vi "HFRR ADV v05.vi"() -> ()   [LabVIEW 2025] (continued)
            n2842 = call "Instrument fgv.vi"("Enum"=T19."READ", "error in (no error) 2"=w3942, "INPUT"=w3940) -> ("error"=w3941:errorcluster, "output"=w3932:T13)  [unwired: 6 in, 1 out]
            n2843 = Bundle By Name(cluster=w3932, "String 36"="String") -> (w3931:T13)
            n2844 = case shown="True" "Write S" {
              selector: "Write S" -> [_ w3962]
              tunnel: w3941 -> [w3955 w3961]
              tunnel: [w3955 w3960] -> w3928
              tunnel: w3931 -> [w3954 w3957]
              tunnel: [w3954 w3956] -> w3927
              frame False {
              }
              frame True {
                n2845 = Not(x=w3962) -> (.not. x?=w3958:bool)
                n2846 = local write "Write S"(w3958) -> ()
                n2847 = call "Instrument fgv.vi"("Enum"=T19."MANUAL WRITE", "error in (no error) 2"=w3961, "INPUT"=w3957) -> ("error"=w3960:errorcluster, "output"=w3956:T13)  [unwired: 6 in, 1 out]
              }
            }
            n2848 = Array Size(array="WriteHumidity") -> (size(s)=w3925:i32)
            n2849 = Greater Than 0?(x=w3925) -> (x > 0?=w3923:bool)
            n2850 = call "Instrument fgv.vi"("Enum"=T19."WRITE", "error in (no error) 2"=w3928, "WriteCC1"="WriteHumidity", "INPUT"=w3927) -> ("error"=w3938:errorcluster, "WriteCC1 2"=w3926:string[], "output"=w3937:T13)  [unwired: 5 in]
            n2851 = case shown="True" w3923 {
              tunnel: w3926 -> [_ w3944]
              frame False {
              }
              frame True {
                n2852 = local write "WriteHumidity"(w3944) -> ()
              }
            }
            n2853 = case shown="Error" w3938 {
              selector: w3938 -> [w3945 w3948]
              tunnel: w3937 -> [w3946 w3953]
              tunnel: [w3946 w3952] -> w3935
              tunnel: [w3945 w3950] -> w3936
              frame No Error {
              }
              frame Error {
                n2854 = call <vilib>:"Clear Errors.vi"("error in (no error)"=w3948) -> ("error out"=w3947:errorcluster)  [unwired: 5 in, 1 out]
                n2855 = call "Instrument fgv.vi"("Enum"=T19."ERROR INIT", "error in (no error) 2"=w3947, "INPUT"=w3953) -> ("error"=w3951:errorcluster, "output"=w3952:T13)  [unwired: 6 in, 1 out]
                n2856 = call <vilib>:"Clear Errors.vi"("error in (no error)"=w3951) -> ("error out"=w3950:errorcluster)  [unwired: 5 in, 1 out]
              }
            }
            n2857 = Unbundle By Name(w3935) -> ("LastCom"=→"LastCom":string, "Read Heave and Surge"=→"Read Humidity":string)
          }
        }
        n2858 = Divide(x="Surge PPR", y="Surge Pitch") -> (x/y=→"Surge Pulses/mm":dbl)
        n2859 = Unbundle By Name(w3910) -> ("Heave COM Status 2"=w3912:bool, "Heave COM Status"=w3911:bool, "Error Heave"=w3908:errorcluster, "Bytes at Heave Port"=→"Bytes at Humidity Port":dbl)
        n2860 = Unbundle By Name(w3908) -> ("status"=→"Humidity Port":bool)
        n2861 = local write "Error Heave"(w3908) -> ()
        n2862 = Not(x=w3911) -> (.not. x?=w3896:bool)
        n2863 = Not(x=w3912) -> (.not. x?=w3897:bool)
        n2864 = local write "Instrument Status"(w3896) -> ()
        n2865 = local write "Heave COM Status 2"(w3897) -> ()
        n2866 = local read "Quit"() -> (w3889:bool)
        n2867 = Select(t=enum16{"init", "MAIN", "Panel Close"}."Panel Close", s=w3889, f=enum16{"init", "MAIN", "Panel Close"}."MAIN") -> (s? t:f=w3888:enum16{"init", "MAIN", "Panel Close"})
      }
      frame "Panel Close" {
      }
      frame Default {
      }
    }
  }
  n2868 = while {
    stop <- w3994 stop-if-true
    n2869 = local read "Read Humidity"() -> (w3972:string)
    n2870 = call <vilib>:"High Resolution Polling Wait.vi"("seconds to wait"=0.1) -> ()  [unwired: 10 in, 1 out]
    n2871 = String Length(string=w3972) -> (length=w3974:i32)
    n2872 = Less?(x=w3974, y=31 ("length")) -> (x < y?=w3970:bool)
    n2873 = case shown="False" w3970 {
      tunnel: w3972 -> [w3995 _]
      tunnel: [w3995 w3996] -> w3971
      frame False {
        "Read Humidity 2" <- w3995
      }
      frame True {
        n2874 = local read "Read Humidity 2"() -> (w3996:string)
      }
    }
    n2875 = Spreadsheet String To Array(delimiter (Tab)=",", format string="", spreadsheet string=w3971, array type (2D Dbl)=string[] []) -> (array=w3989:string[])
    n2876 = for {
      tunnel: w3989 -> [w3999] mode=indexing
      tunnel: string[] ["STATE;", "SET;", "RH;", "T;", "AMB_RH;", "AMB_T;", "PUMP;", "FAN_IN;", "FAN_OUT;", "DEHUM;", "CURRENT;", "STALL;"] -> [w3998] mode=indexing
      tunnel: [w3997] -> w3988 mode=indexing
      n2877 = Match Pattern(string=w3999, regular expression=w3998) -> (after substring=w3997:string)  [unwired: 1 in, 3 out]
    }
    n2878 = Index Array(array=w3988) -> (element #1=→"STATE :":string, element #2=→"SET :":string, element #3=w3977:string, element #4=→"T :":string, element #5=w3969:string, element #6=→"AMB_T :":string, element #7=→"PUMP :":string, element #8=→"FAN_IN :":string, element #9=→"FAN_OUT :":string, element #10=→"DEHUM :":string, element #11=→"CURRENT :":string, element #12=→"STALL :":string)  [unwired: 12 in]
    "RH :" <- w3977
    "AMB_RH :" <- w3969
    n2879 = Fract/Exp String To Number(string=w3977) -> (number=→"RH Numeric:":dbl)  [unwired: 3 in, 1 out]
    n2880 = Fract/Exp String To Number(string=w3969) -> (number=w3968:dbl)  [unwired: 3 in, 1 out]
    n2881 = local write "Ambient Humidity :"(w3968) -> ()
    n2882 = local read "Quit"() -> (w3994:bool)
  }
  n2883 = disable-structure shown="Disabled" {
    frame Disabled {
      n2884 = while {
        tunnel: [w4233] -> _
        i -> [w4233]
        stop <- w4230 stop-if-true
        n2885 = local read "powstat"() -> (w4231:bool)
        n2886 = case shown="True" w4231 {
          frame False {
          }
          frame True {
            n2887 = local read "RUN"() -> (w4234:bool)
            n2888 = case shown="True" w4234 {
              frame False {
                w4264 = 65.0 ("y")
                n2889 = local read "Set Hz"() -> (w4292:dbl)
                n2890 = local read "NORMAL LOAD"() -> (w4293:dbl)
                n2891 = Multiply(x=w4292, y=60.0) -> (x*y=w4299:dbl)
                n2892 = Multiply(x=1.2 ("y"), y=0.949) -> (x*y=w4268:dbl)
                n2893 = Multiply(x=1.2 ("y"), y=0.8166) -> (x*y=w4272:dbl)
                n2894 = Multiply(x=1.2 ("y"), y=0.851) -> (x*y=w4267:dbl)
                n2895 = local read "FF 2"() -> (w4291:dbl)
                n2896 = Absolute Value(x=w4299) -> (abs(x)=w4297:dbl)
                n2897 = local read "Stroke"() -> (w4266:dbl)
                n2898 = Less?(x=w4266, y=w4272) -> (x < y?=w4269:bool)
                n2899 = In Range and Coerce(upper limit=w4268, x=w4266, lower limit=w4267) -> (In Range?=w4270:bool)  [unwired: 1 out]
                n2900 = case shown="13.." w4291 {
                  tunnel: [1 2 3] -> w4289
                  frame 0..10, Default {
                    # "Normal"
                  }
                  frame 11, 12 {
                  }
                  frame 13.. {
                  }
                }
                "FF STATE" <- w4289
                n2901 = local read "TEMP"() -> (w4252:dbl)
                n2902 = case shown="3601.." w4297 {
                  tunnel: [1 2 3] -> w4295
                  frame 0..3000, Default {
                    # "Normal"
                  }
                  frame 3001..3600 {
                  }
                  frame 3601.. {
                  }
                }
                n2903 = case shown="11.." w4293 {
                  tunnel: [1 3] -> w4294
                  frame 1..10, Default {
                  }
                  frame 11.. {
                  }
                }
                "NL STATE" <- w4294
                n2904 = Multiply(x=1.2 ("y"), y=0.95) -> (x*y=w4282:dbl)
                n2905 = Multiply(x=w4264, y=0.954) -> (x*y=w4256:dbl)
                n2906 = Or(x=w4269, y=w4270) -> (x .or. y?=w4271:bool)
                n2907 = Greater Or Equal?(x=w4266, y=w4282) -> (x >= y?=w4279:bool)
                n2908 = Multiply(x=w4264, y=0.99) -> (x*y=w4253:dbl)
                n2909 = Greater Or Equal?(x=w4252, y=w4253) -> (x >= y?=w4258:bool)
                n2910 = Greater Or Equal?(x=w4252, y=w4256) -> (x >= y?=w4255:bool)
                n2911 = case shown="0, 1, Default" w4266 {
                  tunnel: [1 3] -> w4283
                  frame 0, 1, Default {
                  }
                  frame 2.. {
                  }
                }
                n2912 = case shown="True" w4279 {
                  tunnel: [1 3] -> w4284
                  frame False {
                  }
                  frame True {
                  }
                }
                n2913 = case shown="True" w4271 {
                  tunnel: [1 2] -> w4285
                  frame False {
                  }
                  frame True {
                  }
                }
                n2914 = case shown="..0" w4252 {
                  tunnel: [2 3 3 1] -> w4259
                  frame 61, 62 {
                  }
                  frame 63.. {
                  }
                  frame ..0 {
                  }
                  frame 10..60, Default {
                  }
                }
                n2915 = case shown="True" w4258 {
                  tunnel: [1 3] -> w4260
                  frame False {
                  }
                  frame True {
                  }
                }
                n2916 = Number To Decimal String(number=w4295) -> (decimal integer string=w4296:string)  [unwired: 1 in]
                n2917 = case shown="True" w4255 {
                  tunnel: [1 2] -> w4261
                  frame False {
                  }
                  frame True {
                  }
                }
                n2918 = Number To Decimal String(number=1) -> (decimal integer string=→"Air temp":string)  [unwired: 1 in]
                n2919 = Number To Decimal String(number=w4289) -> (decimal integer string=→"ff_st":string)  [unwired: 1 in]
                n2920 = local write "sp_st"(w4296) -> ()
                n2921 = Number To Decimal String(number=w4294) -> (decimal integer string=→"nl_st":string)  [unwired: 1 in]
                n2922 = Build Array(w4259, w4260, w4261) -> (w4262:i32[])
                n2923 = Build Array(w4283, w4284, w4285) -> (w4286:i32[])
                n2924 = Array Max & Min(array=w4262) -> (max value=w4263:i32)  [unwired: 3 out]
                n2925 = Array Max & Min(array=w4286) -> (max value=w4287:i32)  [unwired: 3 out]
                n2926 = Number To Decimal String(number=w4263) -> (decimal integer string=w4251:string)  [unwired: 1 in]
                n2927 = Number To Decimal String(number=w4287) -> (decimal integer string=→"Stroke Ln 2":string)  [unwired: 1 in]
                n2928 = local write "temp_st"(w4251) -> ()
              }
              frame True {
                w4349 = 65.0 ("y")
                # "Healthy -1\nWarning -2\nError -3"
                n2929 = local read "TEMP"() -> (w4360:dbl)
                n2930 = local read "NORMAL LOAD"() -> (w4364:dbl)
                n2931 = local read "Set Hz"() -> (w4362:dbl)
                n2932 = Multiply(x=1.2 ("y"), y=0.949) -> (x*y=w4344:dbl)
                n2933 = Multiply(x=1.2 ("y"), y=0.8166) -> (x*y=w4340:dbl)
                n2934 = Multiply(x=1.2 ("y"), y=0.851) -> (x*y=w4345:dbl)
                n2935 = Multiply(x=w4349, y=0.954) -> (x*y=w4356:dbl)
                n2936 = Multiply(x=w4349, y=0.99) -> (x*y=w4359:dbl)
                n2937 = Greater Or Equal?(x=w4360, y=w4359) -> (x >= y?=w4354:bool)
                n2938 = Multiply(x=w4362, y=60.0) -> (x*y=w4368:dbl)
                n2939 = Greater Or Equal?(x=w4360, y=w4356) -> (x >= y?=w4357:bool)
                n2940 = local read "FF 2"() -> (w4363:dbl)
                n2941 = local read "Stroke"() -> (w4346:dbl)
                n2942 = Less?(x=w4346, y=w4340) -> (x < y?=w4343:bool)
                n2943 = In Range and Coerce(upper limit=w4344, x=w4346, lower limit=w4345) -> (In Range?=w4342:bool)  [unwired: 1 out]
                n2944 = Absolute Value(x=w4368) -> (abs(x)=w4366:dbl)
                n2945 = case shown="63.." w4360 {
                  tunnel: [2 3 3 1] -> w4353
                  frame 61, 62 {
                  }
                  frame 63.. {
                  }
                  frame ..0 {
                  }
                  frame 10..60, Default {
                  }
                }
                n2946 = case shown="True" w4354 {
                  tunnel: [1 3] -> w4352
                  frame False {
                  }
                  frame True {
                  }
                }
                n2947 = case shown="True" w4357 {
                  tunnel: [1 2] -> w4351
                  frame False {
                  }
                  frame True {
                  }
                }
                n2948 = Multiply(x=1.2 ("y"), y=0.95) -> (x*y=w4330:dbl)
                n2949 = case shown="1..10, Default" w4364 {
                  tunnel: [1 3] -> w4371
                  frame 1..10, Default {
                  }
                  frame 11.. {
                  }
                }
                n2950 = case shown="0..10, Default" w4363 {
                  tunnel: [1 2 3] -> w4370
                  frame 0..10, Default {
                  }
                  frame 11, 12 {
                  }
                  frame 13.. {
                  }
                }
                n2951 = case shown="3601.." w4366 {
                  tunnel: [1 2 3] -> w4365
                  frame 0..3000, Default {
                    # "Normal"
                  }
                  frame 3001..3600 {
                  }
                  frame 3601.. {
                  }
                }
                n2952 = Or(x=w4343, y=w4342) -> (x .or. y?=w4341:bool)
                n2953 = Greater Or Equal?(x=w4346, y=w4330) -> (x >= y?=w4333:bool)
                n2954 = case shown="0, 1, Default" w4346 {
                  tunnel: [1 3] -> w4329
                  frame 0, 1, Default {
                  }
                  frame 2.. {
                  }
                }
                n2955 = case shown="True" w4333 {
                  tunnel: [1 3] -> w4328
                  frame False {
                  }
                  frame True {
                  }
                }
                n2956 = case shown="True" w4341 {
                  tunnel: [1 2] -> w4327
                  frame False {
                  }
                  frame True {
                  }
                }
                n2957 = Build Array(w4353, w4352, w4351) -> (w4350:i32[])
                n2958 = Number To Decimal String(number=w4365) -> (decimal integer string=→"sp_st":string)  [unwired: 1 in]
                n2959 = Array Max & Min(array=w4350) -> (max value=w4347:i32)  [unwired: 3 out]
                "TEMP STATE" <- w4347
                n2960 = Number To Decimal String(number=w4371) -> (decimal integer string=w4374:string)  [unwired: 1 in]
                n2961 = Number To Decimal String(number=w4370) -> (decimal integer string=w4372:string)  [unwired: 1 in]
                n2962 = Number To Decimal String(number=w4347) -> (decimal integer string=→"temp_st":string)  [unwired: 1 in]
                n2963 = Build Array(w4329, w4328, w4327) -> (w4326:i32[])
                n2964 = local write "nl_st"(w4374) -> ()
                n2965 = local write "ff_st"(w4372) -> ()
                n2966 = Number To Decimal String(number=1) -> (decimal integer string=w4369:string)  [unwired: 1 in]
                n2967 = Array Max & Min(array=w4326) -> (max value=w4325:i32)  [unwired: 3 out]
                n2968 = local write "Air temp"(w4369) -> ()
                n2969 = Number To Decimal String(number=w4325) -> (decimal integer string=w4324:string)  [unwired: 1 in]
                n2970 = local write "Stroke Ln 2"(w4324) -> ()
              }
            }
            n2971 = local read "Stroke Ln 2"() -> (w4236:string)
            n2972 = local read "nl_st"() -> (w4242:string)
            n2973 = local read "ff_st"() -> (w4239:string)
            n2974 = local read "sp_st"() -> (w4240:string)
            n2975 = local read "temp_st"() -> (w4241:string)
            n2976 = local read "Air temp"() -> (w4235:string)
            n2977 = Replace Array Subset(array="in", new element #1=w4242, index #1=1 ("index"), new element #2=w4239, index #2=2 ("index"), new element #3=w4241, index #3=3 ("index"), new element #4=w4240, index #4=4 ("index"), new element #5=w4236, index #5=5 ("index"), new element #6=w4235, index #6=6 ("index"), new element #7="Sensor State" ("new element/subarray"), index #7=0 ("index")) -> (→"out":string[])
          }
        }
        n2978 = Wait (ms)(milliseconds to wait=u32 10) -> ()  [unwired: 1 out]
        n2979 = local read "Quit"() -> (w4230:bool)
      }
      n2980 = while {
        stop <- w4205 stop-if-true
        n2981 = local read "run replace"() -> (w4207:bool)
        n2982 = Wait (ms)(milliseconds to wait=u32 100) -> ()  [unwired: 1 out]
        n2983 = Equal?(x="FLAG 2", y=0.0) -> (x = y?=w4208:bool)
        n2984 = case shown="True" w4208 {
          frame False {
          }
          frame True {
            n2985 = local write "FLAG 2"(100.0 ("FLAG 2")) -> ()
            n2986 = call <vilib>:"Read Characters From File.vi"("file path (dialog if empty)"=path "C:/LAB-IQ-NXT/WO 2449 TT.sig", "convert eol? (no:F)"=FALSE ("append to file? (new file:F)")) -> ("character string"=w4211:string)  [unwired: 4 in, 3 out]
            n2987 = call <vilib>:"Read Characters From File.vi"("file path (dialog if empty)"=path "C:/LAB-IQ-NXT/WO 2449 TRH.sig", "convert eol? (no:F)"=FALSE ("append to file? (new file:F)")) -> ("character string"=w4212:string)  [unwired: 4 in, 3 out]
            n2988 = Decimal String To Number(string=w4211) -> (number=w4213:i32)  [unwired: 2 in, 1 out]
            n2989 = local write "Total No. of Tests"(w4213) -> ()
            n2990 = Decimal String To Number(string=w4212) -> (number=w4216:i32)  [unwired: 2 in, 1 out]
            n2991 = local write "SEN.RUN HRS"(w4216) -> ()
          }
        }
        n2992 = case shown="True" w4207 {
          frame False {
          }
          frame True {
            n2993 = Equal?(x="FLAG 4", y=0.0) -> (x = y?=w4220:bool)
            n2994 = case shown="False" w4220 {
              frame False {
                n2995 = Get Date/Time In Seconds() -> (seconds since 1Jan1904=w4226:timestamp)
                n2996 = local read "START 3"() -> (w4224:dbl)
                n2997 = To Double Precision Float(number=w4226) -> (double precision float=w4225:dbl)
                n2998 = Subtract(x=w4225, y=w4224) -> (x-y=→"SENSOR TIME":dbl)
              }
              frame True {
                n2999 = Get Date/Time In Seconds() -> (seconds since 1Jan1904=w4228:timestamp)
                n3000 = local write "FLAG 4"(100.0 ("FLAG")) -> ()
                n3001 = To Double Precision Float(number=w4228) -> (double precision float=→"START 3":dbl)
              }
            }
          }
        }
        n3002 = local read "Quit"() -> (w4205:bool)
      }
      n3003 = while {
        shift-right: [w4005] -> _
        shift-left: _ -> [w4006]
        tunnel: [w4001] -> _
        i -> [w4001]
        stop <- w4000 stop-if-true
        n3004 = Wait (ms)(milliseconds to wait=u32 50 ("Refresh Rate (ms)")) -> ()  [unwired: 1 out]
        n3005 = local read "Json End Flg"() -> (w4002:bool)
        n3006 = Not(x="Upld AR 2") -> ()  [unwired: 1 out]
        n3007 = local read "Upld AR 2"() -> (w4003:bool)
        n3008 = call "Elapsed Time9"("Time Target (s)"="Sen.Upload Rate (s)", "Reset"=FALSE, "Auto Reset"=TRUE) -> ("Time has Elapsed"=w4012:bool)  [unwired: 9 in, 7 out]
        n3009 = Or(x=w4012, y=w4002) -> (x .or. y?=w4008:bool)
        n3010 = case shown="True" w4008 {
          frame False {
          }
          frame True {
            w4104 = "\"SensorName\":\"" ("string")
            w4074 = " \"},{"
            w4099 = "\",\"SensorState\":\""
            w4101 = "\",\"SensorModelNumber\":\"" ("string")
            w4100 = "\",\"SensorRuntimeHours\":\"" ("string")
            n3011 = local read "model num"() -> (w4098:string[])
            n3012 = local read "Sensor name"() -> (w4117:string[])
            n3013 = local read "run"() -> (w4088:string[])
            n3014 = local read "SENSOR TIME"() -> (w4044:dbl)
            n3015 = local read "out"() -> (w4037:string[])
            n3016 = local read "Total No. of Tests"() -> (w4042:dbl)
            n3017 = Select(t=60.0, s="Run test 3", f=3600.0) -> (s? t:f=w4052:dbl)
            n3018 = Index Array(array=w4098, index #1=1 ("index")) -> (element #1=w4097:string, element #2=w4096:string, element #3=w4095:string, element #4=w4094:string, element #5=w4093:string, element #6=w4092:string)  [unwired: 5 in]
            n3019 = Index Array(array=w4088, index #1=1 ("index")) -> (element #1=w4087:string, element #2=w4086:string, element #3=w4085:string, element #4=w4084:string, element #5=w4083:string, element #6=w4082:string)  [unwired: 5 in]
            n3020 = Index Array(array=w4117, index #1=1 ("index")) -> (element #1=w4116:string, element #2=w4115:string, element #3=w4114:string, element #4=w4113:string, element #5=w4103:string, element #6=w4102:string)  [unwired: 5 in]
            n3021 = Index Array(array=w4037, index #1=1 ("index")) -> (element #1=w4069:string, element #2=w4068:string, element #3=w4067:string, element #4=w4066:string, element #5=w4065:string, element #6=w4064:string)  [unwired: 5 in]
            n3022 = local read "SEN.RUN HRS"() -> (w4040:dbl)
            n3023 = Divide(x=w4044, y=w4052) -> (x/y=w4051:dbl)
            n3024 = Increment(x=w4051) -> (x+1=w4047:dbl)
            n3025 = Number To Decimal String(number=w4047) -> (decimal integer string=→"run hrs":string)  [unwired: 1 in]
            n3026 = Divide(x=w4040, y=3600.0 ("f")) -> (x/y=w4035:dbl)
            n3027 = Round To Nearest(number=w4035) -> (nearest integer value=w4033:dbl)
            n3028 = Number To Decimal String(number=w4033) -> (decimal integer string=w4034:string)  [unwired: 1 in]
            n3029 = Number To Decimal String(number=w4042) -> (decimal integer string=w4043:string)  [unwired: 1 in]
            n3030 = local read "Model No"() -> (w4048:string)
            n3031 = local read "UUID"() -> (w4143:string)
            n3032 = local read "Serial No"() -> (w4147:string)
            n3033 = local read "Secret Key"() -> (w4148:string)
            n3034 = Concatenate Strings("\",\"MachineSerialNumber\":\"" ("string"), w4147) -> (w4151:string)
            n3035 = Concatenate Strings("\",\"ModelNumber\":\"" ("string"), w4048) -> (w4049:string)
            n3036 = Concatenate Strings("\",\"MachineRuntimeHours\":\"" ("string"), w4034) -> (w4152:string)
            n3037 = Concatenate Strings("\",\"MachineRuntimeCycles\":\"", w4043) -> (w4145:string)
            n3038 = Concatenate Strings(w4101, w4097) -> (w4131:string)
            n3039 = Concatenate Strings(w4100, w4087) -> (w4132:string)
            n3040 = Concatenate Strings(w4099, w4069) -> (w4130:string)
            n3041 = Concatenate Strings(w4151, w4049, w4152, w4145) -> (w4154:string)
            n3042 = Concatenate Strings(w4101, w4096) -> (w4128:string)
            n3043 = Concatenate Strings(w4100, w4086) -> (w4127:string)
            n3044 = Concatenate Strings(w4099, w4068) -> (w4129:string)
            n3045 = Concatenate Strings(w4101, w4095) -> (w4123:string)
            n3046 = Concatenate Strings(w4100, w4085) -> (w4124:string)
            n3047 = Concatenate Strings(w4099, w4067) -> (w4122:string)
            n3048 = Concatenate Strings(w4101, w4094) -> (w4120:string)
            n3049 = Concatenate Strings(w4100, w4084) -> (w4119:string)
            n3050 = Concatenate Strings(w4099, w4066) -> (w4121:string)
            n3051 = Concatenate Strings(w4131, w4132, w4130) -> (w4133:string)
            n3052 = Concatenate Strings(w4101, w4093) -> (w4110:string)
            n3053 = Concatenate Strings(w4100, w4083) -> (w4111:string)
            n3054 = Concatenate Strings(w4101, w4092) -> (w4107:string)
            n3055 = Concatenate Strings(w4100, w4082) -> (w4106:string)
            n3056 = Concatenate Strings(w4099, w4065) -> (w4109:string)
            n3057 = Concatenate Strings(w4099, w4064) -> (w4108:string)
            n3058 = Concatenate Strings("{\"SecretKey\":\"", w4148, w4154, "\",\"UUID\" : \"", w4143, "\",\"SensorInformation\":", "[{" ("string")) -> (w4081:string)
            n3059 = Concatenate Strings(w4128, w4127, w4129) -> (w4126:string)
            n3060 = Concatenate Strings(w4123, w4124, w4122) -> (w4125:string)
            n3061 = Concatenate Strings(w4120, w4119, w4121) -> (w4118:string)
            n3062 = Concatenate Strings(w4110, w4111, w4109) -> (w4112:string)
            n3063 = Concatenate Strings(w4107, w4106, w4108) -> (w4105:string)
            n3064 = Concatenate Strings(w4104, w4116, w4133, w4074) -> (w4080:string)
            n3065 = Concatenate Strings(w4104, w4115, w4126, w4074) -> (w4079:string)
            n3066 = Concatenate Strings(w4104, w4114, w4125, w4074) -> (w4078:string)
            n3067 = Concatenate Strings(w4104, w4113, w4118, w4074) -> (w4077:string)
            n3068 = Concatenate Strings(w4104, w4103, w4112, w4074) -> (w4076:string)
            n3069 = Concatenate Strings(w4104, w4102, w4105, "\"}" ("string")) -> (w4075:string)
            n3070 = Concatenate Strings(w4081, w4080, w4079, w4078, w4077, w4076, w4075, "]}" ("string")) -> (w4072:string)
            n3071 = local read "SEN.RUN HRS"() -> (w4039:dbl)
            n3072 = disable-structure shown="Disabled" {
              frame Disabled {
                n3073 = local read "state"() -> (w4158:string[])
                n3074 = Delete From Array(array=w4158, index=0) -> (array with subset deleted=w4156:string[])  [unwired: 1 in, 1 out]
                n3075 = for {
                  N: 6 -> [_]
                  tunnel: w4156 -> [w4169] mode=indexing
                  tunnel: [w4168] -> w4155 mode=indexing
                  n3076 = Equal?(x=w4169, y="Warning") -> (x = y?=w4165:bool)
                  n3077 = Equal?(x=w4169, y="Healthy") -> (x = y?=w4162:bool)
                  n3078 = Select(t="2" ("y"), s=w4165, f="3" ("y")) -> (s? t:f=w4160:string)
                  n3079 = Select(t="1" ("y"), s=w4162, f=w4160) -> (s? t:f=w4168:string)
                }
                "state1" <- w4155
              }
              frame Enabled {
              }
            }
            n3080 = stacked-sequence {
              tunnel: w4072 -> [w4180 _ _]
              tunnel: [_ _ w4196] -> _
              frame #0 {
                (unwired) FALSE ("convert eol (F)")
                w4182 = enum16{"start", "end", "current"}."start" ("pos mode (0:2)")
                n3081 = local read "Path"() -> (w4176:path)
                n3082 = Path To String(path=w4176) -> (string=w4188:string)
                n3083 = Concatenate Strings(w4188, "\\", "Sensor File Name") -> (w4189:string)
                n3084 = local write "standard output 2"(" ") -> ()
                n3085 = String To Path(string=w4189) -> (path=w4179:path)
                n3086 = call <vilib>:"Open_Create_Replace File.vi"("advisory dialog? (display:T)"=FALSE, "function (open:0)"=T20."create or replace", "file path"=w4179) -> ("error out"=w4192:errorcluster, "refnum"=w4191:refnum<file>)  [unwired: 5 in, 2 out]
                n3087 = Set File Position(refnum=w4191, from (0:start)=w4182, error in=w4192) -> (refnum out=w4172:refnum<file>, error out=w4171:errorcluster)  [unwired: 1 in]
                n3088 = Write to Binary File(file (use dialog)=w4172, data=" ", error in=w4171, 5:FALSE ("prepend array or string size? (T)")) -> (refnum out=w4183:refnum<file>, error out=w4184:errorcluster)  [unwired: 2 in, 1 out]
                n3089 = Set File Position(offset (in bytes) (0)=w4182, refnum=w4183, error in=w4184) -> (refnum out=w4175:refnum<file>, error out=w4174:errorcluster)  [unwired: 1 in]
                n3090 = Write to Binary File(file (use dialog)=w4175, data=w4180, error in=w4174, 5:FALSE ("prepend array or string size? (T)")) -> (error out=w4178:errorcluster)  [unwired: 2 in, 2 out]
                n3091 = flat-sequence {
                  tunnel: w4179 -> [w4194]
                  tunnel: w4178 -> [_]
                  frame #0 {
                    n3092 = call <vilib>:"Read Characters From File.vi"("file path (dialog if empty)"=w4194) -> ("character string"=→"Sensor Health JSON string":string)  [unwired: 5 in, 3 out]
                  }
                }
                "SinglePoint  2" <- w4180
              }
              frame #1 {
              }
              frame #2 {
                (unwired) "\"Stored\": true" ("string")
                n3093 = call <vilib>:"System Exec.vi"("run minimized? (F)"=TRUE, "wait until completion? (T)"=TRUE, "working directory"=path "C:/LAB-IQ-NXT", "command line"="C:\\LAB-IQ-NXT\\JPostH.bat") -> ("standard error"=→"Respose From Server 2":string, "standard output"=w4199:string)  [unwired: 4 in, 2 out]
                "standard output 2" <- w4199
                n3094 = Match Pattern(string=w4199, regular expression="JSONH Check String") -> (match substring=w4197:string, offset past match=w4196:i32)  [unwired: 1 in, 2 out]
                n3095 = Equal?(x=w4197, y="JSONH Check String") -> (x = y?=→"Upload \nConfirmed 2":bool)
              }
            }
            n3096 = Divide(x=w4039, y=3600.0 ("f")) -> (x/y=w4032:dbl)
            n3097 = local read "run time"() -> (w4089:string[])
            n3098 = Round To Nearest(number=w4032) -> (nearest integer value=w4031:dbl)
            n3099 = Number To Decimal String(number=w4031) -> (decimal integer string=w4030:string)  [unwired: 1 in]
            n3100 = Index Array(array="Sensor Information", index (col) #1=0 ("disabled index (col)"), index (col) #2=1 ("index (col)"), index (col) #3=2 ("index (col)"), index (col) #4=3 ("index (col)")) -> (element #1=→"Sensor name":string[], element #2=→"model num":string[], element #3=→"run time":string[], element #4=→"state":string[])  [unwired: 4 in]
            n3101 = Insert Into Array(array=w4089, index=1, new element #1=w4030, new element #2=w4030, new element #3=w4030, new element #4=w4030, new element #5=w4030, new element #6=w4030) -> (w4054:string[])
            "run" <- w4054
            n3102 = local read "out"() -> (w4036:string[])
            n3103 = local read "Sensor Information"() -> (w4056:string[][])
            n3104 = Replace Array Subset(array=w4056, new element #1=w4054, index (col) #1=2 ("disabled index (col)"), new element #2=w4036, index (col) #2=3 ("index (col)")) -> (w4055:string[][])  [unwired: 2 in]
            n3105 = local write "Sensor Information"(w4055) -> ()
          }
        }
        n3106 = case shown="True" w4003 {
          frame False {
          }
          frame True {
            n3107 = Equal?(x="FLAG", y=0.0) -> (x = y?=w4020:bool)
            n3108 = case shown="False" w4020 {
              frame False {
                n3109 = Get Date/Time In Seconds() -> (seconds since 1Jan1904=w4026:timestamp)
                n3110 = local read "START 2"() -> (w4024:dbl)
                n3111 = To Double Precision Float(number=w4026) -> (double precision float=w4025:dbl)
                n3112 = Subtract(x=w4025, y=w4024) -> (x-y=→"SENSOR TIME  2":dbl)
              }
              frame True {
                n3113 = Get Date/Time In Seconds() -> (seconds since 1Jan1904=w4028:timestamp)
                n3114 = To Double Precision Float(number=w4028) -> (double precision float=→"START 2":dbl)
                n3115 = local write "FLAG"(100.0 ("FLAG")) -> ()
              }
            }
          }
        }
        n3116 = disable-structure shown="Disabled" {
          disable-tunnel: w4006 -> [w4015 _]
          disable-tunnel: [w4014 _] -> w4005
          frame Disabled {
            n3117 = local read "Json St Flg"() -> (w4013:bool)
            n3118 = case shown="True" w4013 {
              tunnel: w4015 -> [w4016 w4018]
              tunnel: [w4016 w4017] -> w4014
              frame False {
              }
              frame True {
                n3119 = Increment(x=w4018) -> (x+1=w4017:dbl)
                "T cycle" <- w4017
                n3120 = local write "Json St Flg"(FALSE ("Json St Flg")) -> ()
              }
            }
          }
          frame Enabled {
          }
        }
        n3121 = local read "Quit"() -> (w4000:bool)
      }
    }
    frame Enabled {
    }
  }
  n3122 = stacked-sequence {
    tunnel: [w4398] -> w18
    frame #0 {
      w4398 = FALSE ("Upload \nConfirmed")
      n3123 = local write "Upload \nConfirmed"(w4398) -> ()
      n3124 = local write "St Str"("") -> ()
    }
  }
  n3125 = disable-structure shown="Disabled" {
    disable-tunnel: w18 -> [w4399 _]
    frame Disabled {
      n3126 = case shown="True" {
        selector: _ -> [_ _]
        tunnel: w4399 -> [_ w4400]
        frame False {
        }
        frame True {
          n3127 = while {
            tunnel: [w4406] -> _
            tunnel: w4400 -> [_]
            i -> [w4406]
            stop <- w4401 stop-if-true
            n3128 = local read "Json End Flg"() -> (w4405:bool)
            n3129 = Wait (ms)(milliseconds to wait=u32 20 ("Refresh Rate (ms)")) -> ()  [unwired: 1 out]
            n3130 = local read "refresh flag"() -> (w4402:bool)
            n3131 = local read "RUN"() -> (w4403:bool)
            n3132 = And(x=w4403, y=w4402) -> (x .and. y?=w4404:bool)
            n3133 = Or(x=w4404, y=w4405) -> (x .or. y?=w4407:bool)
            "AR Led" <- w4407
            n3134 = case shown="True" w4407 {
              frame False {
              }
              frame True {
                w4424 = "\",\""
                n3135 = local read "UUID"() -> (w4422:string)
                n3136 = local write "refresh flag"(FALSE ("refresh flag")) -> ()
                n3137 = local read "time"() -> (w4411:dbl)
                n3138 = Multiply(x=w4411, y=60.0) -> (x*y=w4410:dbl)
                n3139 = Concatenate Strings("UUID\" : \"", w4422, "\"}") -> (w4425:string)
                n3140 = Number To Fractional String(number=w4410, width (-)=i16 10, precision (6)=i16 4) -> (F-format string=w4439:string)  [unwired: 1 in]
                n3141 = Concatenate Strings("{", "\"Time\":\"", w4439, w4424) -> (w4434:string)
                n3142 = stacked-sequence {
                  tunnel: w4424 -> [w4487 w4495 w4502 w4510 w4518 w4527 w4534]
                  tunnel: [w4488 _ _ _ _ _ _] -> w4438
                  tunnel: [_ w4496 _ _ _ _ _] -> w4437
                  tunnel: [_ _ w4503 _ _ _ _] -> w4436
                  tunnel: [_ _ _ w4512 _ _ _] -> w4435
                  tunnel: w4425 -> [_ _ _ _ _ _ w4545]
                  tunnel: [_ _ _ _ _ _ w4544] -> w4421
                  tunnel: [_ _ _ _ _ w4524 _] -> w4420
                  tunnel: [_ _ _ _ w4517 _ _] -> w4419
                  frame #0 {
                    n3143 = local read "NORMAL LOAD"() -> (w4486:dbl)
                    n3144 = Number To Fractional String(number=w4486, width (-)=i16 10, precision (6)=i16 4) -> (F-format string=w4489:string)  [unwired: 1 in]
                    n3145 = Concatenate Strings("NormalLoad\":\"", w4489, w4487) -> (w4488:string)
                  }
                  frame #1 {
                    n3146 = local read "Temp"() -> (w4494:dbl)
                    n3147 = Number To Fractional String(number=w4494, width (-)=i16 10, precision (6)=i16 4) -> (F-format string=w4497:string)  [unwired: 1 in]
                    n3148 = Concatenate Strings("Temperature\":\"", w4497, w4495) -> (w4496:string)
                  }
                  frame #2 {
                    n3149 = local read "cof"() -> (w4500:dbl)
                    n3150 = Number To Fractional String(number=w4500, width (-)=i16 10, precision (6)=i16 4) -> (F-format string=w4504:string)  [unwired: 1 in]
                    n3151 = Concatenate Strings("FrictionalForce\":\"", w4504, w4502) -> (w4503:string)
                  }
                  frame #3 {
                    n3152 = local read "Set Hz"() -> (w4508:dbl)
                    n3153 = Multiply(x=w4508, y=60.0) -> (x*y=w4507:dbl)
                    n3154 = Number To Fractional String(number=w4507, width (-)=i16 10, precision (6)=i16 4) -> (F-format string=w4513:string)  [unwired: 1 in]
                    n3155 = Concatenate Strings("Speed\":\"", w4513, w4510) -> (w4512:string)
                  }
                  frame #4 {
                    n3156 = local read "Stroke Ln"() -> (w4516:dbl)
                    n3157 = Number To Fractional String(number=w4516, width (-)=i16 10, precision (6)=i16 4) -> (F-format string=w4520:string)  [unwired: 1 in]
                    n3158 = Concatenate Strings("LinearDeformation\":\"", w4520, w4518) -> (w4517:string)
                  }
                  frame #5 {
                    n3159 = local read "AIR TEMP"() -> (w4523:dbl)
                    n3160 = local read "Json St Flg"() -> (w4525:bool)
                    n3161 = local read "Json End Flg"() -> (w4526:bool)
                    n3162 = Number To Fractional String(number=w4523, width (-)=i16 10, precision (6)=i16 4) -> (F-format string=w4529:string)  [unwired: 1 in]
                    n3163 = Concatenate Strings("Vibration\":\"", w4529, w4527) -> (w4524:string)
                    n3164 = And(x=w4525, y=w4526) -> ()  [unwired: 1 out]
                  }
                  frame #6 {
                    n3165 = local read "Json End Flg"() -> (w4533:bool)
                    n3166 = Get Date/Time In Seconds() -> (seconds since 1Jan1904=w4541:timestamp)
                    n3167 = local read "Json St Flg"() -> (w4532:bool)
                    n3168 = To Double Precision Float(number=w4541) -> (double precision float=w4540:dbl)
                    n3169 = Subtract(x=w4540, y=2082844800.0) -> (x-y=w4538:dbl)
                    n3170 = Number To Fractional String(number=w4538, width (-)=i16 12, precision (6)=i16 0) -> (F-format string=w4535:string)  [unwired: 1 in]
                    n3171 = case shown="True" w4533 {
                      tunnel: ["" w4548] -> w4542
                      tunnel: w4535 -> [_ w4549]
                      tunnel: w4534 -> [_ w4547]
                      frame False {
                      }
                      frame True {
                        n3172 = local write "Json End Flg"(FALSE ("Json St Flg")) -> ()
                        n3173 = Concatenate Strings("End\": \"", w4549, w4547) -> (w4548:string)
                      }
                    }
                    n3174 = case shown="True" w4532 {
                      tunnel: [w4552 w4555] -> w4543
                      tunnel: w4535 -> [_ w4556]
                      tunnel: w4534 -> [_ w4553]
                      frame False {
                        n3175 = local read "St Str"() -> (w4552:string)
                      }
                      frame True {
                        n3176 = Concatenate Strings("Start\":\"", w4556, w4553) -> (w4555:string)
                        "St Str" <- w4555
                        n3177 = local write "Json St Flg"(FALSE ("Json St Flg")) -> ()
                      }
                    }
                    n3178 = Concatenate Strings(w4543, w4542, w4545) -> (w4544:string)
                  }
                }
                n3179 = local read "FILE"() -> (w4413:string)
                n3180 = Concatenate Strings("\",\"OperatorID\":\"" ("string"), "Operator ID") -> (w4416:string)
                n3181 = Concatenate Strings("\",\"DatasetTitle\":\"" ("string"), w4413) -> (w4415:string)
                n3182 = Concatenate Strings("\",\"SerialNumber\":\"" ("string"), "Serial No") -> (w4445:string)
                n3183 = Concatenate Strings("\",\"ModelNumber\":\"" ("string"), "Model No") -> (w4444:string)
                n3184 = Concatenate Strings(w4445, w4444) -> (w4427:string)
                n3185 = Concatenate Strings("{\"SecretKey\":\"", "Secret Key", w4427, w4416, w4415, "\",\"Samples\":[") -> (w4432:string)
                n3186 = Concatenate Strings(w4434, w4438, w4437, w4436, w4435, w4419, w4420, w4421) -> (w4433:string)
                n3187 = Concatenate Strings(w4432, w4433, "]}") -> (w4431:string)
                n3188 = stacked-sequence {
                  tunnel: w4431 -> [w4460 _ _]
                  tunnel: [_ _ w4477] -> _
                  frame #0 {
                    (unwired) FALSE ("convert eol (F)")
                    w4462 = enum16{"start", "end", "current"}."start" ("pos mode (0:2)")
                    n3189 = Path To String(path="Path") -> (string=w4468:string)
                    n3190 = Concatenate Strings(w4468, "\\", "Data File Name") -> (w4470:string)
                    n3191 = local write "standard output"(" ") -> ()
                    n3192 = String To Path(string=w4470) -> (path=w4459:path)
                    n3193 = call <vilib>:"Open_Create_Replace File.vi"("advisory dialog? (display:T)"=FALSE, "function (open:0)"=T20."create or replace", "file path"=w4459) -> ("error out"=w4473:errorcluster, "refnum"=w4472:refnum<file>)  [unwired: 5 in, 2 out]
                    n3194 = Set File Position(refnum=w4472, from (0:start)=w4462, error in=w4473) -> (refnum out=w4453:refnum<file>, error out=w4452:errorcluster)  [unwired: 1 in]
                    n3195 = Write to Binary File(file (use dialog)=w4453, data=" ", error in=w4452, 5:FALSE ("prepend array or string size? (T)")) -> (refnum out=w4463:refnum<file>, error out=w4464:errorcluster)  [unwired: 2 in, 1 out]
                    n3196 = Set File Position(offset (in bytes) (0)=w4462, refnum=w4463, error in=w4464) -> (refnum out=w4456:refnum<file>, error out=w4455:errorcluster)  [unwired: 1 in]
                    n3197 = Write to Binary File(file (use dialog)=w4456, data=w4460, error in=w4455, 5:FALSE ("prepend array or string size? (T)")) -> (error out=w4458:errorcluster)  [unwired: 2 in, 2 out]
                    n3198 = flat-sequence {
                      tunnel: w4459 -> [w4475]
                      tunnel: w4458 -> [_]
                      frame #0 {
                        n3199 = call <vilib>:"Read Characters From File.vi"("file path (dialog if empty)"=w4475) -> ("character string"=→"JSON string":string)  [unwired: 5 in, 3 out]
                      }
                    }
                    "SinglePoint" <- w4460
                  }
                  frame #1 {
                  }
                  frame #2 {
                    (unwired) "\"Stored\": true" ("string")
                    n3200 = call <vilib>:"System Exec.vi"("run minimized? (F)"=TRUE, "wait until completion? (T)"=TRUE, "working directory"=path "C:/LAB-IQ-NXT", "command line"="C:\\LAB-IQ-NXT\\JPost.bat") -> ("standard error"=→"Respose From Server":string, "standard output"=w4480:string)  [unwired: 4 in, 2 out]
                    "standard output" <- w4480
                    n3201 = Match Pattern(string=w4480, regular expression="JSON Check String") -> (match substring=w4478:string, offset past match=w4477:i32)  [unwired: 1 in, 2 out]
                    n3202 = Equal?(x=w4478, y="JSON Check String") -> (x = y?=→"Upload \nConfirmed":bool)
                  }
                }
              }
            }
            n3203 = local read "Quit"() -> (w4401:bool)
          }
        }
      }
    }
    frame Enabled {
    }
  }
  n3204 = disable-structure shown="Disabled" {
    disable-tunnel: w17 -> [w4563 _]
    frame Disabled {
      n3205 = while {
        shift-right: [w4571] -> w4559
        shift-left: _ -> [w4572]
        shift-right: [w4569] -> w4560
        shift-left: errorcluster {"status"=TRUE, "code"=0, "source"="Init"} ("error out") -> [w4570]
        shift-right: [w4567] -> _
        shift-left: "" -> [w4568]
        tunnel: [w4565] -> _
        tunnel: w4563 -> [_]
        i -> [w4565]
        stop <- w4564 stop-if-true
        n3206 = flat-sequence {
          tunnel: [w4573] -> w4566
          frame #0 {
            n3207 = Wait (ms)(milliseconds to wait=10.0 ("Delay")) -> (millisecond timer value=w4573:u32)
          }
        }
        n3208 = case shown="No Error" w4570 {
          selector: w4570 -> [w4606 w4728]
          tunnel: [w4588 w4730] -> w4571
          tunnel: [w4587 w4729] -> w4569
          tunnel: w4572 -> [w4607 w4722]
          tunnel: w4568 -> [w4586 w4721]
          tunnel: [w4585 w4721] -> w4567
          tunnel: w4566 -> [_ _]
          frame No Error {
            n3209 = Concatenate Strings("COMMAND", "\r", "\n") -> (w4597:string)
            n3210 = case shown="True" "Measure" {
              tunnel: w4607 -> [w4633 w4640]
              tunnel: w4606 -> [w4632 w4639]
              tunnel: [w4633 w4638] -> w4605
              tunnel: [w4632 w4637] -> w4584
              tunnel: w4597 -> [_ w4636]
              frame False {
              }
              frame True {
                n3211 = VISA Write(VISA resource name=w4640, write buffer=w4636, error in (no error)=w4639) -> (VISA resource name out=w4638:refnum<visa-resource-name>, error out=w4637:errorcluster)  [unwired: 1 out]
                n3212 = local write "Read String"("") -> ()
                n3213 = local write "Measure"(FALSE) -> ()
              }
            }
            n3214 = property class="Instr"(reference=w4605, error in=w4584) -> (reference out=w4604:refnum<visa-resource-name>, error out=w4603:errorcluster, "Serial Settings:Number of Bytes at Serial Port"=w4602:u32)
            n3215 = Greater?(x=w4602, y=u32 100) -> (0:w4600:bool)
            n3216 = case shown="True" w4600 {
              tunnel: w4604 -> [w4643 w4668]
              tunnel: w4603 -> [w4642 w4667]
              tunnel: w4602 -> [_ w4666]
              tunnel: [w4643 w4665] -> w4590
              tunnel: [w4642 w4664] -> w4589
              tunnel: w4586 -> [w4641 w4663]
              tunnel: [w4641 ""] -> w4585
              frame False {
              }
              frame True {
                w4653 = u32 6 ("y")
                # "Page 84 of \nmanual"
                n3217 = VISA Read(VISA resource name=w4668, byte count=w4666, error in (no error)=w4667) -> (VISA resource name out=w4665:refnum<visa-resource-name>, read buffer=w4661:string, error out=w4664:errorcluster)  [unwired: 1 out]
                n3218 = while {
                  tunnel: w4661 -> [w4717]
                  tunnel: [w4713] -> w4655 mode=indexing
                  tunnel: [w4707] -> w4659 mode=indexing
                  tunnel: [w4705] -> _
                  i -> [w4705]
                  stop <- w4710 stop-if-true
                  n3219 = String Subset(string=w4717, offset (0)=w4705) -> (substring=w4712:string)  [unwired: 1 in]
                  n3220 = String To Byte Array(string=w4712) -> (unsigned byte array=w4716:u8[])
                  n3221 = String Length(string=w4712) -> (length=w4711:i32)
                  n3222 = Index Array(array=w4716) -> (element=w4715:u8)  [unwired: 1 in]
                  n3223 = Equal To 0?(x=w4711) -> (x = 0?=w4710:bool)
                  n3224 = Number To Boolean Array(number=w4715) -> (Boolean array=w4709:bool[])
                  n3225 = Reverse 1D Array(array=w4709) -> (reversed array=w4708:bool[])
                  n3226 = And(x=w4709, y=bool[] [FALSE, FALSE, FALSE, FALSE, FALSE, FALSE, TRUE, TRUE] ("Boolean array")) -> (x .and. y?=w4713:bool[])
                  n3227 = And(x=w4708, y=bool[] [FALSE, FALSE, TRUE, TRUE, TRUE, TRUE, TRUE, TRUE] ("Boolean array")) -> (x .and. y?=w4707:bool[])
                }
                n3228 = Concatenate Strings(w4663, w4661) -> (→"Read String":string)
                n3229 = while {
                  tunnel: w4655 -> [w4704] mode=indexing
                  tunnel: [w4700] -> w4658
                  i -> [w4700]
                  stop <- w4701 stop-if-true
                  n3230 = Search 1D Array(1D array=w4704, element=TRUE) -> (index of element=w4702:i32)  [unwired: 1 in]
                  n3231 = Less Than 0?(x=w4702) -> (x < 0?=w4701:bool)
                }
                n3232 = Delete From Array(array=w4659, length=w4658, index (row)=0) -> (array with subset deleted=w4654:bool[][])  [unwired: 1 in, 1 out]
                n3233 = Array Size(array=w4654) -> (size(s)=w4656:i32[])
                n3234 = Index Array(array=w4656) -> (element=w4648:i32)  [unwired: 1 in]
                n3235 = Greater?(x=w4648, y=w4653) -> (0:w4651:bool)
                n3236 = Subtract(x=w4648, y=w4653) -> (x-y=w4652:u32)
                n3237 = Select(t=w4652, s=w4651, f=u32 0) -> (s? t:f=w4649:u32)
                n3238 = while {
                  tunnel: w4654 -> [w4687]
                  tunnel: [w4689] -> w4647 mode=indexing
                  tunnel: w4649 -> [w4671]
                  i -> [w4688]
                  stop <- w4686 stop-if-true
                  w4678 = 6 ("index")
                  w4677 = 2 ("length")
                  # "Page 65 of \nmanual"
                  n3239 = Multiply(x=u32 3 ("y"), y=w4688) -> (x*y=w4685:u32)
                  n3240 = Divide(x=u32 102 ("y"), y=u32 65520) -> (x/y=w4695:dbl)
                  n3241 = Greater Or Equal?(x=w4685, y=w4671) -> (x >= y?=w4686:bool)
                  n3242 = Index Array(array=w4687, index (row) #1=w4685) -> (element #1=w4683:bool[], element #2=w4682:bool[], element #3=w4681:bool[])  [unwired: 5 in]
                  n3243 = Reverse 1D Array(array=w4683) -> (reversed array=w4676:bool[])
                  n3244 = Reverse 1D Array(array=w4682) -> (reversed array=w4680:bool[])
                  n3245 = Reverse 1D Array(array=w4681) -> (reversed array=w4679:bool[])
                  n3246 = Delete From Array(array=w4676, length=w4677, index=w4678) -> (array with subset deleted=w4672:bool[])  [unwired: 1 out]
                  n3247 = Delete From Array(array=w4680, length=w4677, index=w4678) -> (array with subset deleted=w4673:bool[])  [unwired: 1 out]
                  n3248 = Delete From Array(array=w4679, length=w4677, index=w4678) -> (array with subset deleted=w4674:bool[])  [unwired: 1 out]
                  n3249 = Insert Into Array(array=bool[] [] ("Boolean array"), new element #1=w4672, new element #2=w4673, new element #3=w4674) -> (w4675:bool[])  [unwired: 1 in]
                  n3250 = Boolean Array To Number(Boolean array=w4675) -> (number=w4684:u32)
                  n3251 = Multiply(x=w4695, y=w4684) -> (x*y=w4694:dbl)
                  n3252 = Decrement(x=w4694) -> (x-1=w4693:dbl)
                  n3253 = Divide(x=w4693, y=u32 100) -> (x/y=w4691:dbl)
                  n3254 = Multiply(x=w4691, y=u32 10) -> (x*y=w4689:dbl)
                }
                n3255 = Delete From Array(array=w4647) -> (array with subset deleted=w4646:dbl[])  [unwired: 2 in, 1 out]
                "Waveform Graph 5" <- w4646
                "Waveform Chart 3" <- w4646
                n3256 = call-poly <vilib>:"Mean.vi"("X"=w4646) -> ("mean"=w4645:dbl)  [unwired: 1 out]
                "Measure_LDS" <- w4645
                n3257 = case shown="True" "Zero 4" {
                  tunnel: w4645 -> [_ w4670]
                  frame False {
                  }
                  frame True {
                    n3258 = local write "Zero 4"(FALSE ("Zero 4")) -> ()
                    "z_measure" <- w4670
                  }
                }
              }
            }
            n3259 = local read "Measure_LDS"() -> (w4580:dbl)
            n3260 = local read "Disp (mm)"() -> (w4579:dbl)
            n3261 = local read "Boolean 7"() -> (w4578:bool)
            n3262 = local read "Boolean 8"() -> (w4577:bool)
            n3263 = case shown="True" "Boolean 8" {
              tunnel: w4579 -> [_ w4610]
              tunnel: w4580 -> [_ w4609]
              frame False {
              }
              frame True {
                n3264 = local read "Captured Values 2"() -> (w4613:dbl[][])
                n3265 = Build Array(w4610, w4609) -> (w4608:dbl[])
                n3266 = Build Array (concatenate)(w4613, w4608) -> (w4611:dbl[][])
                n3267 = local write "Captured Values 2"(w4611) -> ()
                n3268 = local write "Boolean 8"(FALSE ("Boolean 8")) -> ()
              }
            }
            n3269 = call "Build XY Graph"("Enable"=w4577, "Reset"=w4578, "Y Input"=w4580, "X Input"=w4579) -> ("XY Graph"=→"?":cluster{"Y":dbl[], "Y":dbl[]}[])  [unwired: 6 in, 1 out]
            n3270 = case shown="True" "Boolean 9" {
              frame False {
              }
              frame True {
                n3271 = local read "Captured Values 2"() -> (w4615:dbl[][])
                n3272 = Index Array(array=w4615, index (col) #1=0 ("disabled index (col)"), index (col) #2=1 ("index (col)")) -> (element #1=w4618:dbl[], element #2=w4617:dbl[])  [unwired: 2 in]
                n3273 = call <vilib>:"Linear Fit.vi"("Y"=w4618, "X"=w4617) -> ("slope"=→"Slope":dbl, "intercept"=→"Intercept":dbl)  [unwired: 9 in, 3 out]
                n3274 = local write "Boolean 9"(FALSE ("Boolean 9")) -> ()
              }
            }
            n3275 = case shown="True" "Boolean 7" {
              frame False {
              }
              frame True {
                n3276 = local write "Captured Values 2"(dbl[][] [] ("Captured Values")) -> ()
                n3277 = local write "Boolean 7"(FALSE ("Boolean 7")) -> ()
              }
            }
            n3278 = Concatenate Strings("COMMAND 2", "\r", "\n") -> (w4592:string)
            n3279 = case shown="True" "Measure 2" {
              tunnel: w4590 -> [w4625 w4631]
              tunnel: w4589 -> [w4624 w4630]
              tunnel: [w4625 w4629] -> w4588
              tunnel: [w4624 w4628] -> w4587
              tunnel: w4592 -> [_ w4627]
              frame False {
              }
              frame True {
                n3280 = local write "Measure 2"(FALSE ("WRITE")) -> ()
                n3281 = VISA Write(VISA resource name=w4631, write buffer=w4627, error in (no error)=w4630) -> (VISA resource name out=w4629:refnum<visa-resource-name>, error out=w4628:errorcluster)  [unwired: 1 out]
              }
            }
          }
          frame Error {
            w4720 = u16 10 items=["1.0"=10, "1.5"=15, "2.0"=20] ("stop bits (10: 1 bit)")
            n3282 = Wait (ms)(milliseconds to wait=u32 20) -> ()  [unwired: 1 out]
            n3283 = VISA Close(VISA resource name=w4722, error in (no error)=w4728) -> (error out=w4727:errorcluster)
            n3284 = call <vilib>:"Clear Errors.vi"("error in (no error)"=w4727) -> ("error out"=w4726:errorcluster)  [unwired: 5 in, 1 out]
            n3285 = call-poly "VISA Configure Serial Port"("VISA resource name"="Laser Disp Sensor", "timeout (10sec)"=u32 200, "Enable Termination\nChar (T)"=TRUE ("Enable Termination\nChar (T)"), "baud rate (9600)"=u32 921600, "error in (no error)"=w4726, "stop bits (10: 1 bit)"=w4720) -> ("VISA resource name out"=w4730:refnum<visa-resource-name>, "error out"=w4729:errorcluster)  [unwired: 8 in]
          }
        }
        n3286 = local read "Quit"() -> (w4564:bool)
      }
      n3287 = VISA Close(VISA resource name=w4559, error in (no error)=w4560) -> (error out=w4558:errorcluster)
      n3288 = call <vilib>:"Clear Errors.vi"("error in (no error)"=w4558) -> ()  [unwired: 5 in, 2 out]
    }
    frame Enabled {
    }
  }
  n3289 = disable-structure shown="Disabled" {
    disable-tunnel: w17 -> [w4735 _]
    frame Disabled {
      n3290 = while {
        tunnel: [w4742] -> _
        shift-right: [w4739] -> w4732
        shift-left: _ -> [w4741]
        shift-right: [w4740] -> w4733
        shift-left: errorcluster {"status"=TRUE, "code"=0, "source"="Init"} ("error out") -> [w4738]
        tunnel: w4735 -> [_]
        i -> [w4742]
        stop <- w4736 stop-if-true
        n3291 = flat-sequence {
          tunnel: w4738 -> [w4833]
